vi "resource entries to table.vi"(7 "Sort Type":T4 items=["RIO device", "resource", "input type", "datatype", "reserver"], 8 "error in (no error)":errorcluster, 10 "fpga resources":cluster{"fpga cd":T1, "resource":T2}[](array[cluster]) {"fpga cd" format="%.0x"}) -> (0 "error out":errorcluster, 1 "sorted resource table out":string[][](array[string]), 2 "fpga resources":cluster{"fpga cd":T1, "resource":T2}[](array[cluster]) {"fpga cd" format="%.0x"})   [LabVIEW 2016, in "FPGA RM System Definition API.lvlib"]
uses:
  FPGA RM System Definition API.lvlib
  <vilib>/NI Veristand/Custom Device API/Custom Device Item Ref.ctl
  API/Types/fpga resource.ctl
  API/Types/Channel Type.ctl
  type defs/viz_type.ctl
  UI/visualizer globals.vi
  <vilib>/NI Veristand/Custom Device API/Get Item Property (String).vi
  <vilib>/NI VeriStand/Custom Device API/Custom Device API.lvlib
  Shared/FPGA RM Shared API.lvlib
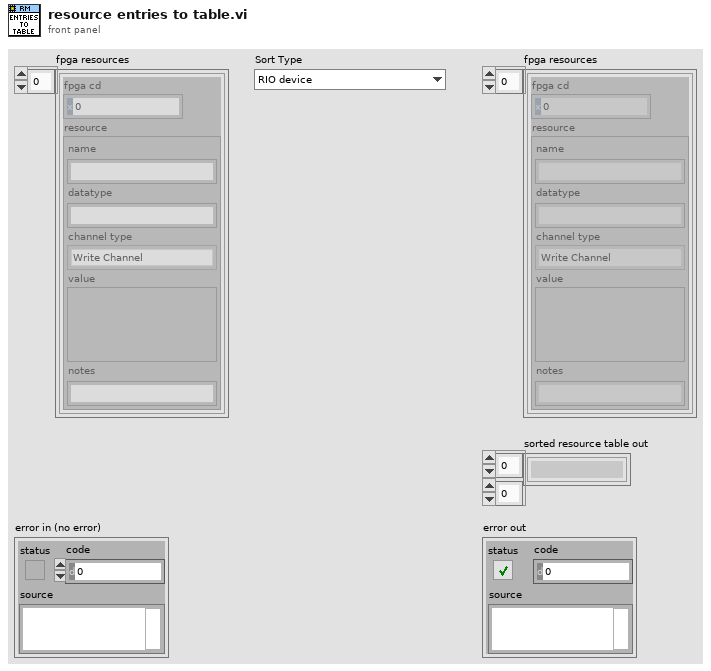
[diagram p1: front panel]
types:
  T1 = typedef "Custom Device API.lvlib/Custom Device Item Ref.ctl" = u64
  T2 = typedef "FPGA RM Shared API.lvlib/fpga resource.ctl" = cluster{"name":string, "datatype":string, "channel type":T3, "value":variant, "notes":string}
  T3 = typedef "FPGA RM Shared API.lvlib/Channel Type.ctl" = enum16{"Write Channel", "Read Channel", "Write Waveform", "Read Waveform"}
  T4 = typedef "FPGA RM System Definition API.lvlib/viz_type.ctl" = u16
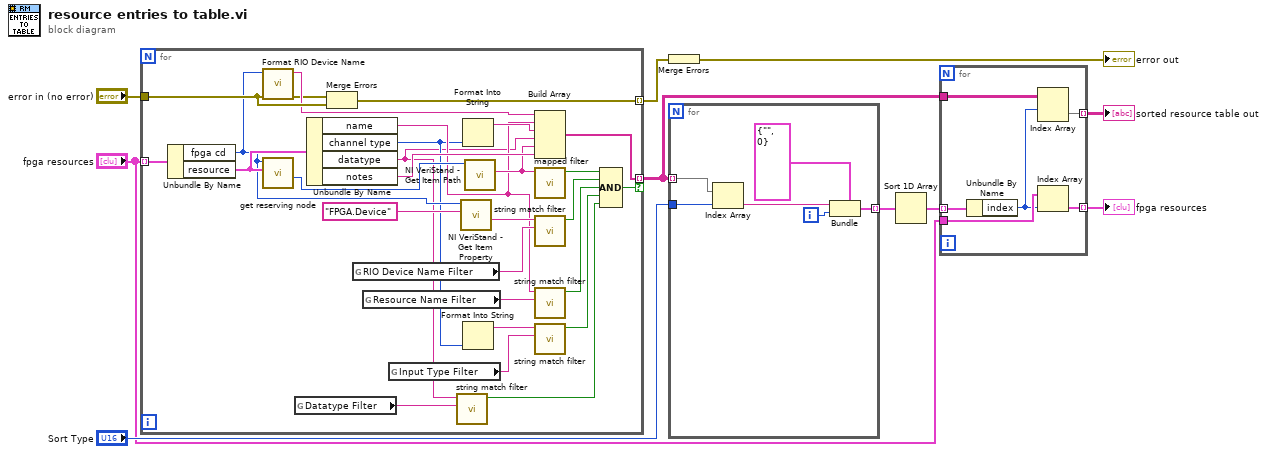
[diagram p0: block diagram]
diagram:
  n1 = for {
    tunnel: "fpga resources" -> [w38] mode=indexing
    tunnel: [w37] -> w3 mode=indexing if=w21
    tunnel: "error in (no error)" -> [w36]
    tunnel: [w35] -> w9 mode=indexing
    n2 = Unbundle By Name(w38) -> ("fpga cd"=w26:T1, "resource"=w32:T2)
    n3 = call "Format RIO Device Name.vi"("error in (no error)"=w36, "FPGA CD Ref"=w26) -> ("error out"=w33:errorcluster, "String"=w34:string)  [unwired: 8 in]
    n4 = call "get reserving node.vi"("FPGA Resource"=w32, "Item Ref in"=w26) -> ("Dependent Node Ref"=w29:T1)  [unwired: 6 in, 3 out]
    n5 = global read "visualizer globals.vi" "Datatype Filter"() -> (w13:string)
    n6 = Unbundle By Name(w32) -> ("name"=w19:string, "channel type"=w17:T3, "datatype"=w12:string, "notes"=w31:string)
    n7 = Merge Errors(w33, w36) -> (w35:errorcluster)
    n8 = global read "visualizer globals.vi" "RIO Device Name Filter"() -> (w24:string)
    n9 = global read "visualizer globals.vi" "Resource Name Filter"() -> (w20:string)
    n10 = global read "visualizer globals.vi" "Input Type Filter"() -> (w15:string)
    n11 = call "string match filter.vi"("string filter value"=w13, "string value"=w12) -> ("match?"=w11:bool)  [unwired: 9 in]
    n12 = call-poly <vilib>:"NI VeriStand - Get Item Property.vi"("Property Name"="FPGA.Device", "Item Ref in"=w26) -> ("Value"=w25:string)  [unwired: 6 in, 3 out]
    n13 = Format Into String(w17) -> (resulting string=w30:string)  [unwired: 3 in, 1 out]
    n14 = Format Into String(w17) -> (resulting string=w16:string)  [unwired: 3 in, 1 out]
    n15 = call <vilib>:"NI VeriStand - Get Item Path.vi"("Item Ref in"=w29) -> ("Path"=w28:string)  [unwired: 7 in, 3 out]
    n16 = Build Array(w34, w19, w30, w12, w28, w31) -> (w37:string[])
    n17 = call "mapped filter.vi"("Path"=w28) -> ("Boolean"=w23:bool)  [unwired: 10 in]
    n18 = call "string match filter.vi"("string filter value"=w24, "string value"=w25) -> ("match?"=w22:bool)  [unwired: 9 in]
    n19 = call "string match filter.vi"("string filter value"=w20, "string value"=w19) -> ("match?"=w18:bool)  [unwired: 9 in]
    n20 = call "string match filter.vi"("string filter value"=w15, "string value"=w16) -> ("match?"=w14:bool)  [unwired: 9 in]
    n21 = Compound Arithmetic op=AND(w23, w22, w18, w14, w11) -> (w21:bool)
  }
  n22 = Merge Errors(w9) -> (→"error out":errorcluster)
  n23 = for {
    tunnel: w3 -> [w41] mode=indexing
    tunnel: "Sort Type" -> [w40]
    tunnel: [w43] -> w6 mode=indexing
    i -> [w44]
    n24 = Index Array(array=w41, index=w40) -> (element=w39:string)
    n25 = Bundle(cluster=cluster{"key":string, "index":i32} {"key"="", "index"=0}, "key"=w39, "index"=w44) -> (w43:cluster{"key":string, "index":i32})
  }
  n26 = Sort 1D Array(array=w6) -> (sorted array=w5:cluster{"key":string, "index":i32}[])
  n27 = for {
    tunnel: w5 -> [w50] mode=indexing
    tunnel: w3 -> [w49]
    tunnel: [w48] -> w4 mode=indexing
    tunnel: "fpga resources" -> [w47]
    tunnel: [w46] -> w1 mode=indexing
    n28 = Unbundle By Name(w50) -> ("index"=w45:i32)
    n29 = Index Array(array=w49, index (row)=w45) -> (element=w48:string[])  [unwired: 1 in]
    n30 = Index Array(array=w47, index=w45) -> (element=w46:cluster{"fpga cd":T1, "resource":T2})
  }
  "sorted resource table out" <- w4
  "fpga resources" <- w1
